vi "Lab16.vi"() -> ()   [LabVIEW 2022 SP3]
uses:
  <vilib>/DAQmx/create/channels.llb/DAQmx Create Channel (CO-Pulse Generation-Frequency).vi
  <vilib>/DAQmx/create/channels.llb/DAQmx Create Channel (CI-Frequency).vi
panel:
  in  "Counter":tag="Dev1/ctr0"
  in  "Divider":dbl=10.0
  in  "Output Terminal":tag="/Dev1/PFI0"
  in  "stop":bool
  in  "Input Terminal":tag="/Dev1/PFI1"
  in  "counter":tag="Dev1/ctr0"
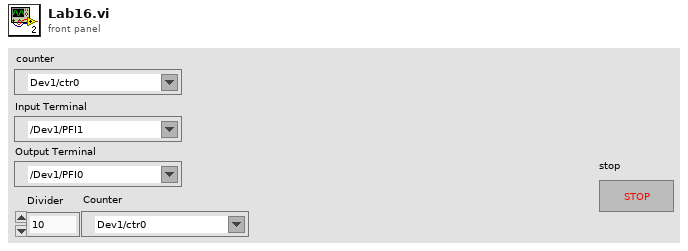
[diagram p1: front panel]
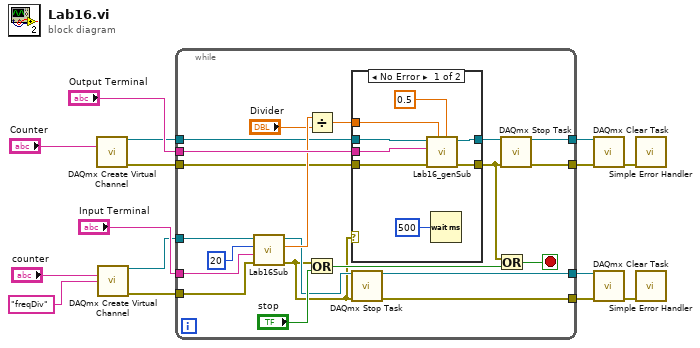
[diagram p0: block diagram]
diagram:
  n1 = call-poly <vilib>:"DAQmx Create Virtual Channel.vi"("counter"="Counter") -> ("task out"=w5:refnum<k21>, "error out"=w4:errorcluster)  [unwired: 13 in]
  n2 = call-poly <vilib>:"DAQmx Create Virtual Channel.vi"("counter"="counter", "name to assign"="freqDiv") -> ("task out"=w7:refnum<k21>, "error out"=w6:errorcluster)  [unwired: 12 in]
  n3 = while {
    tunnel: "Output Terminal" -> [w36]
    tunnel: [w28] -> w13
    tunnel: [w29] -> w12
    tunnel: "Input Terminal" -> [w27]
    tunnel: w7 -> [w26]
    tunnel: w6 -> [w25]
    tunnel: w5 -> [w24]
    tunnel: w4 -> [w23]
    tunnel: [w18] -> w2
    tunnel: [w17] -> w1
    stop <- w32 stop-if-true
    n4 = call "Lab16Sub.vi"("error in (no error)"=w25, "CI.Freq.Term"=w27, "Samples per \nMeasurement"=20 ("Samples per \nMeasurement"), "Refnum in"=w26) -> ("error out"=w19:errorcluster, "Measured Frequency"=w35:dbl, "Refnum out"=w20:refnum<k21>)  [unwired: 5 in]
    n5 = Divide(x=w35, y="Divider") -> (x/y=w33:dbl)
    n6 = Or(x=w19, y="stop") -> (x .or. y?=w21:bool)
    n7 = case shown="No Error" w19 {
      tunnel: w36 -> [w44 _]
      tunnel: w33 -> [w43 _]
      tunnel: [w41 w46] -> w31
      tunnel: [w40 w45] -> w30
      tunnel: w24 -> [w38 w46]
      tunnel: w23 -> [w37 w45]
      frame No Error {
        n8 = call "Lab16_genSub.vi"("duty cycle"=0.5, "frequency"=w43, "error in"=w37, "CO.Pulse.Term"=w44, "task in"=w38) -> ("error out"=w40:errorcluster, "task out"=w41:refnum<k21>)  [unwired: 5 in]
        n9 = Wait (ms)(milliseconds to wait=u32 500) -> ()  [unwired: 1 out]
      }
      frame Error {
      }
    }
    n10 = call <vilib>:"DAQmx Stop Task.vi"("task/channels in"=w20, "error in"=w19) -> ("task out"=w18:refnum<k21>, "error out"=w17:errorcluster)  [unwired: 12 in]
    n11 = Or(x=w30, y=w21) -> (x .or. y?=w32:bool)
    n12 = call <vilib>:"DAQmx Stop Task.vi"("task/channels in"=w31, "error in"=w30) -> ("task out"=w28:refnum<k21>, "error out"=w29:errorcluster)  [unwired: 12 in]
  }
  n13 = call <vilib>:"DAQmx Clear Task.vi"("task in"=w13, "error in"=w12) -> ("error out"=w15:errorcluster)  [unwired: 13 in]
  n14 = call <vilib>:"DAQmx Clear Task.vi"("task in"=w2, "error in"=w1) -> ("error out"=w3:errorcluster)  [unwired: 13 in]
  n15 = call <vilib>:"Simple Error Handler.vi"("error in (no error)"=w15) -> ()  [unwired: 4 in, 5 out]
  n16 = call <vilib>:"Simple Error Handler.vi"("error in (no error)"=w3) -> ()  [unwired: 4 in, 5 out]
